vi "pulsed ODMR Sequence Generator.vi"(0 "N Loop":i32=10000, 1 "Rabi Frequency":dbl, 5 "AOM Pulse length":dbl=2.5e-06, 7 "AOM Rest time":dbl=1e-06, 9 "Signal Delay":dbl=6e-07, 11 "APD signal width":dbl=5e-07, 12 "MW Delay":dbl, 13 "Pulse offset":dbl) -> (4 "Pulse Sequence":T1(array[cluster]))   [LabVIEW 2012]
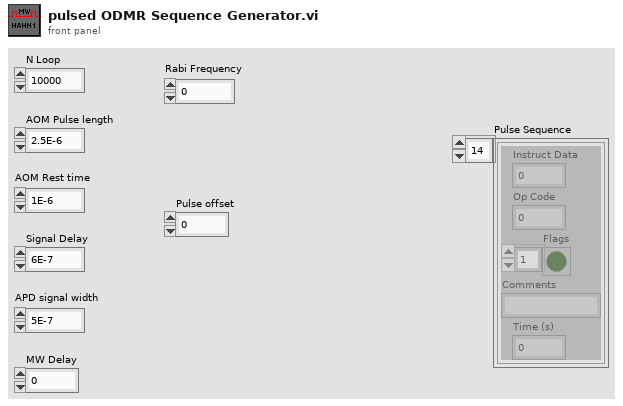
[diagram p1: front panel]
types:
  T1 = cluster{"Instruct Data":i32, "Op Code":i32, "Flags":bool[], "Comments":string, "Time (s)":dbl}[]
  T2 = cluster{"Instruct Data":i32, "Op Code":i32, "Flags":bool[], "Comments":string, "Time (s)":dbl}
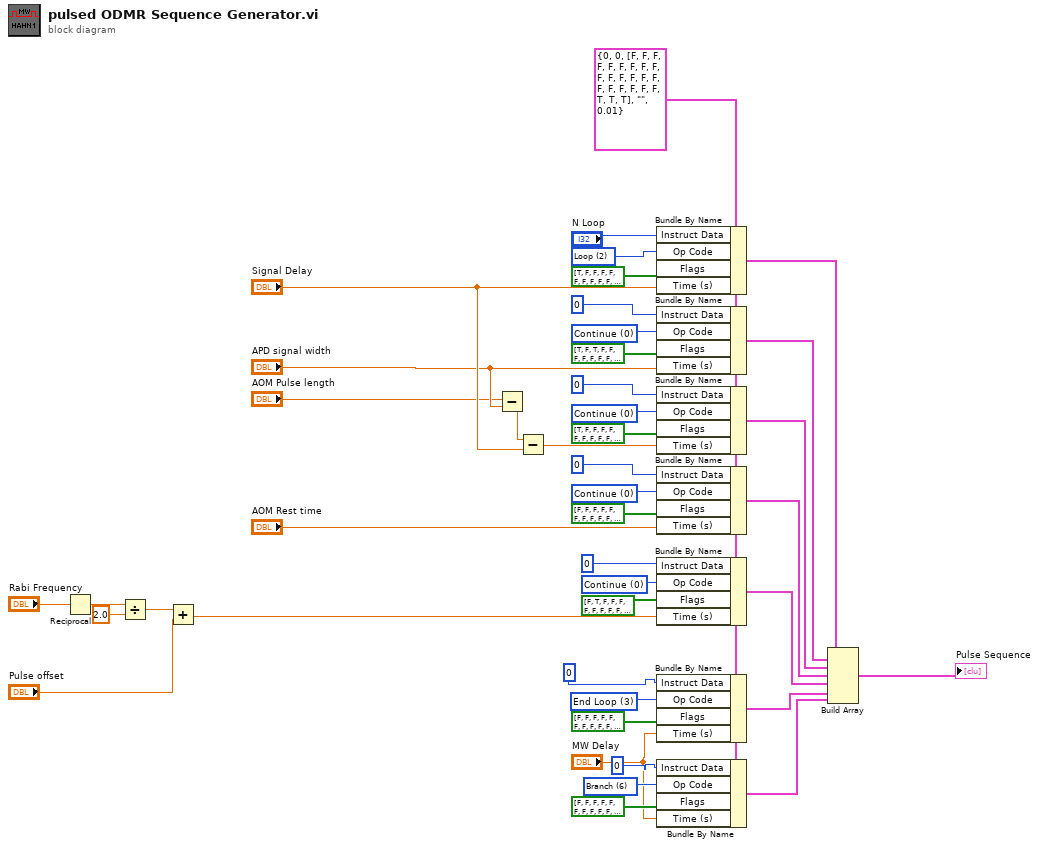
[diagram p0: block diagram]
diagram:
  w8 = 6 items=["Continue", "Stop", "Loop", "End Loop", "JSR", "RTS", "Branch", "Long Delay", "Wait"] ("Op Code")
  w14 = 0 items=["Continue", "Stop", "Loop", "End Loop", "JSR", "RTS", "Branch", "Long Delay", "Wait"] ("Op Code")
  w24 = 3 items=["Continue", "Stop", "Loop", "End Loop", "JSR", "RTS", "Branch", "Long Delay", "Wait"] ("Op Code")
  w29 = 0 items=["Continue", "Stop", "Loop", "End Loop", "JSR", "RTS", "Branch", "Long Delay", "Wait"] ("Op Code")
  w33 = 0 items=["Continue", "Stop", "Loop", "End Loop", "JSR", "RTS", "Branch", "Long Delay", "Wait"] ("Op Code")
  w36 = 0 items=["Continue", "Stop", "Loop", "End Loop", "JSR", "RTS", "Branch", "Long Delay", "Wait"] ("Op Code")
  w38 = 2 items=["Continue", "Stop", "Loop", "End Loop", "JSR", "RTS", "Branch", "Long Delay", "Wait"] ("Op Code")
  w2 = T2 {"Instruct Data"=0, "Op Code"=0, "Flags"=[FALSE, FALSE, FALSE, FALSE, FALSE, FALSE, FALSE, FALSE, FALSE, FALSE, FALSE, FALSE, FALSE, FALSE, FALSE, FALSE, FALSE, FALSE, FALSE, FALSE, FALSE, TRUE, TRUE, TRUE], "Comments"="", "Time (s)"=0.01} ("PB Inst 2")
  n1 = Reciprocal(x="Rabi Frequency") -> (1/x=w18:dbl)
  n2 = Divide(x=w18, y=2.0) -> (x/y=w17:dbl)
  n3 = Add(x=w17, y="Pulse offset") -> (x+y=w10:dbl)
  n4 = Subtract(x="AOM Pulse length", y="APD signal width") -> (x-y=w31:dbl)
  n5 = Subtract(x=w31, y="Signal Delay") -> (x-y=w27:dbl)
  n6 = Bundle By Name(cluster=w2, "Instruct Data"="N Loop", "Op Code"=w38, "Flags"=bool[] [TRUE, FALSE, FALSE, FALSE, FALSE, FALSE, FALSE, FALSE, FALSE, FALSE, FALSE, FALSE, FALSE, FALSE, FALSE, FALSE, FALSE, FALSE, FALSE, FALSE, FALSE, TRUE, TRUE, TRUE], "Time (s)"="Signal Delay") -> (w23:T2)
  n7 = Bundle By Name(cluster=w2, "Instruct Data"=0, "Op Code"=w36, "Flags"=bool[] [TRUE, FALSE, TRUE, FALSE, FALSE, FALSE, FALSE, FALSE, FALSE, FALSE, FALSE, FALSE, FALSE, FALSE, FALSE, FALSE, FALSE, FALSE, FALSE, FALSE, FALSE, TRUE, TRUE, TRUE], "Time (s)"="APD signal width") -> (w22:T2)
  n8 = Bundle By Name(cluster=w2, "Instruct Data"=0, "Op Code"=w33, "Flags"=bool[] [TRUE, FALSE, FALSE, FALSE, FALSE, FALSE, FALSE, FALSE, FALSE, FALSE, FALSE, FALSE, FALSE, FALSE, FALSE, FALSE, FALSE, FALSE, FALSE, FALSE, FALSE, TRUE, TRUE, TRUE], "Time (s)"=w27) -> (w21:T2)
  n9 = Bundle By Name(cluster=w2, "Instruct Data"=0, "Op Code"=w29, "Flags"=bool[] [FALSE, FALSE, FALSE, FALSE, FALSE, FALSE, FALSE, FALSE, FALSE, FALSE, FALSE, FALSE, FALSE, FALSE, FALSE, FALSE, FALSE, FALSE, FALSE, FALSE, FALSE, TRUE, TRUE, TRUE], "Time (s)"="AOM Rest time") -> (w20:T2)
  n10 = Bundle By Name(cluster=w2, "Instruct Data"=0, "Op Code"=w14, "Flags"=bool[] [FALSE, TRUE, FALSE, FALSE, FALSE, FALSE, FALSE, FALSE, FALSE, FALSE, FALSE, FALSE, FALSE, FALSE, FALSE, FALSE, FALSE, FALSE, FALSE, FALSE, FALSE, TRUE, TRUE, TRUE], "Time (s)"=w10) -> (w11:T2)
  n11 = Bundle By Name(cluster=w2, "Instruct Data"=0 ("y"), "Op Code"=w24, "Flags"=bool[] [FALSE, FALSE, FALSE, FALSE, FALSE, FALSE, FALSE, FALSE, FALSE, FALSE, FALSE, FALSE, FALSE, FALSE, FALSE, FALSE, FALSE, FALSE, FALSE, FALSE, FALSE, TRUE, TRUE, TRUE], "Time (s)"="MW Delay") -> (w4:T2)
  n12 = Bundle By Name(cluster=w2, "Instruct Data"=0 ("y"), "Op Code"=w8, "Flags"=bool[] [FALSE, FALSE, FALSE, FALSE, FALSE, FALSE, FALSE, FALSE, FALSE, FALSE, FALSE, FALSE, FALSE, FALSE, FALSE, FALSE, FALSE, FALSE, FALSE, FALSE, FALSE, TRUE, TRUE, TRUE], "Time (s)"="MW Delay") -> (w1:T2)
  n13 = Build Array(w23, w22, w21, w20, w11, w4, w1) -> (→"Pulse Sequence":T1)
